vi "CODCr质控流程 (子VI).vi"(9 "CODCr量程切换":enum32{"H", "L", "AUTO"}(ring)=enum."AUTO", 10 "CODCr":bool) -> (3 "布尔":bool)   [LabVIEW 2016, in "质控单元.lvlib"]
panel:
  out "CODCr中断报警":bool
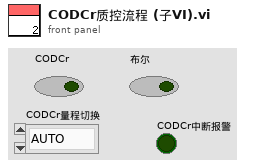
[diagram p1: front panel]
types:
  T1 = enum16{"待机", "启动水样测量", "水样测量中", "启动加标", "启动加标回收", "加标回收测量中", "结束"}
  T2 = cluster{"测量模式":enum16{"水样测量", "标样核查", "零点核查", "跨度核查", "空白测试", "加标回收", "平行样", "校零", "校标"}}
  T3 = enum16{"空闲", "水样测试", "标样核查", "零点核查", "跨度核查", "空白测试", "平行样测试", "加标回收", "空白校准", "标样校准", "初始化（清洗）"}
  T4 = cluster{"系统时间":timestamp, "工作状态":enum16{"空闲", "水样测试", "标样核查", "零点核查", "跨度核查", "空白测试", "平行样测试", "加标回收", "空白校准", "标样校准", "初始化（清洗）"}, "测量模式":enum16{"待机", "连续模式", "周期模式", "定点模式", "受控模式", "手动模式"}, "告警代码":enum16{"无告警", "缺试剂告警", "缺水样告警", "缺蒸馏水告警", "缺标液告警", "仪表漏液告警", "标定异常告警", "超量程告警", "加热异常", "低试剂预警", "超上限告警", "超下限告警", "仪表内部其他异常", "滴定异常告警", "电极异常告警", "量程切换告警", "参数设置告警", "PH电极电位异常", "电导率电极异常", "浊度光度异常", "溶解氧电极异常", "溶解氧光强异常", "温度异常告警", "PH异常告警", "溶解氧异常告警", "电导率异常告警", "浊度异常告警", "叶绿素异常告警", "藻密度异常告警", "蓝绿藻异常告警", "ORP异常告警", "氨氮异常告警", "清洁刷异常告警", "SD卡异常告警", "蓝牙异常告警", "Wifi异常告警", "流程异常告警"}, "故障代码":enum16{"无故障", "电机故障", "温度故障", "通讯故障", "滴定故障"}, "日志代码":u16, "软件版本":u16, "F0":sgl, "F1":sgl, "F2":sgl, "F3":sgl, "T":sgl, "H":sgl, "id":u16, "flowid":u16, "量程":u16, "总磷控温温度1":sgl, "营养盐控温温度2":sgl, "ADC":sgl}
  T5 = cluster{"因子编码":u32, "单位":u16, "标样参考值":sgl, "水样数据时间":timestamp, "水样实测值":sgl, "水样数据标识":string, "标样数据时间":timestamp, "标样实测值":sgl, "标样数据标识":string, "空白数据时间":timestamp, "空白实测值":sgl, "空白数据标识":string, "零点核查数据时间":timestamp, "零点核查实测值":sgl, "零点核查数据标识":string, "跨度核查数据时间":timestamp, "跨度核查实测值":sgl, "跨度核查数据标识":string, "加标回收数据时间":timestamp, "加标回收实测值":sgl, "加标回收数据标识":string, "平行样数据时间":timestamp, "平行样实测值":sgl, "平行样数据标识":string}
  T6 = cluster{"量程":dbl, "检出限":dbl, "加标前水样浓度":dbl, "加标后水样浓度":dbl, "加标水杯定容体积":dbl, "加标母液浓度":dbl, "加标体积":dbl, "加标回收率":dbl}
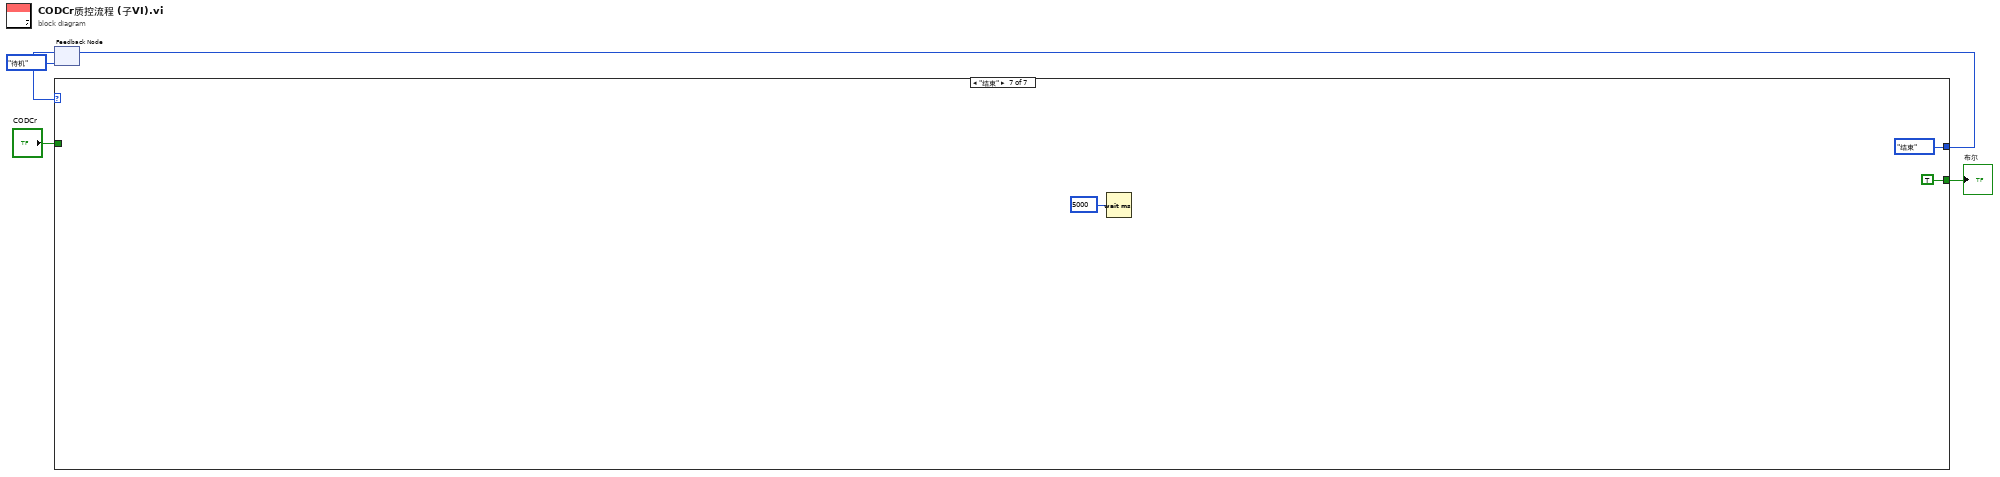
[diagram p0: block diagram]
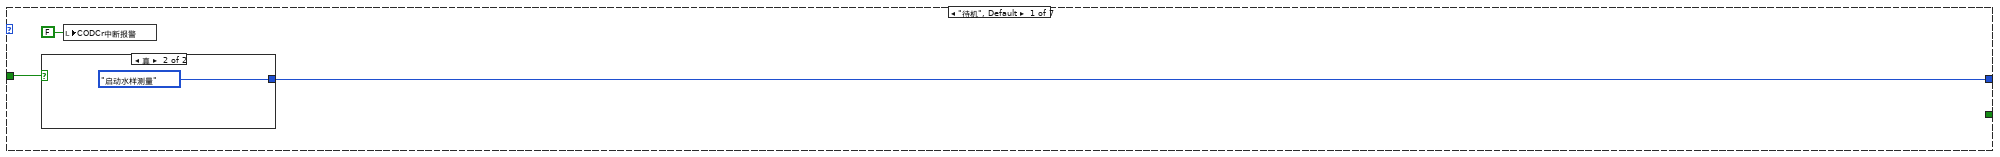
[diagram p2: hidden frame]
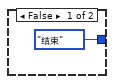
[diagram p3: hidden frame]
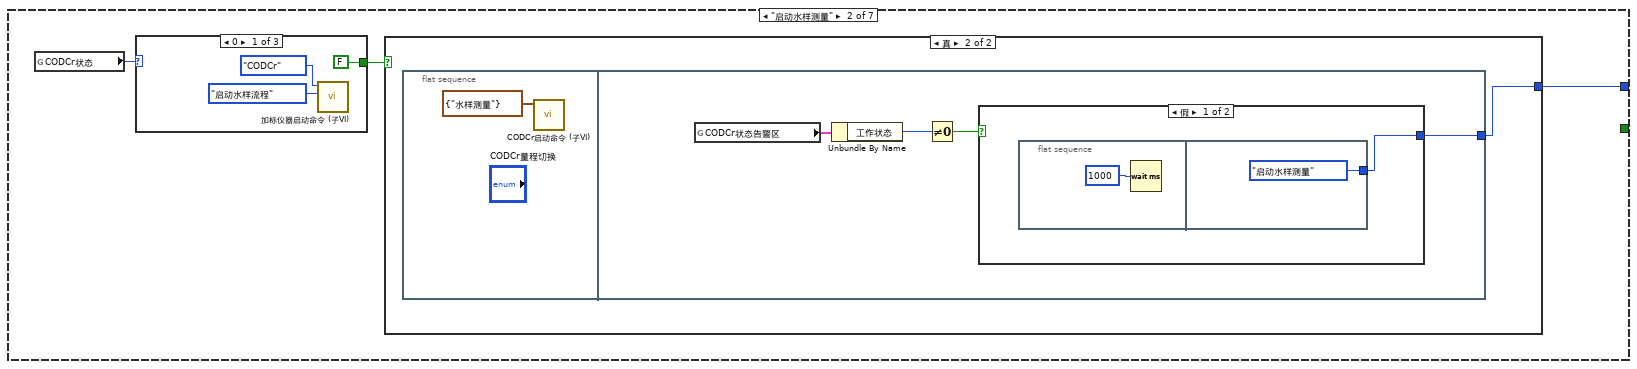
[diagram p4: hidden frame]
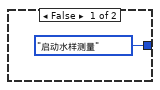
[diagram p5: hidden frame]
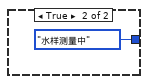
[diagram p6: hidden frame]
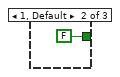
[diagram p7: hidden frame]
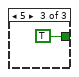
[diagram p8: hidden frame]
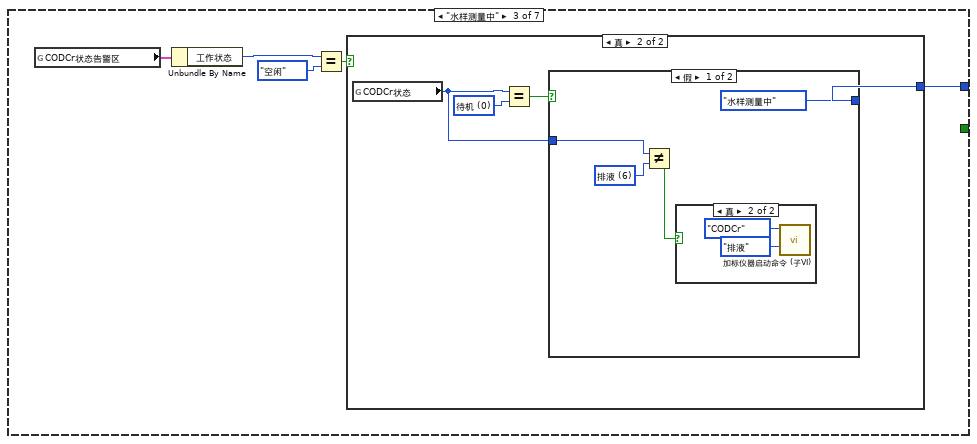
[diagram p9: hidden frame]
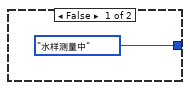
[diagram p10: hidden frame]
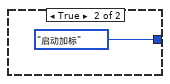
[diagram p12: hidden frame]
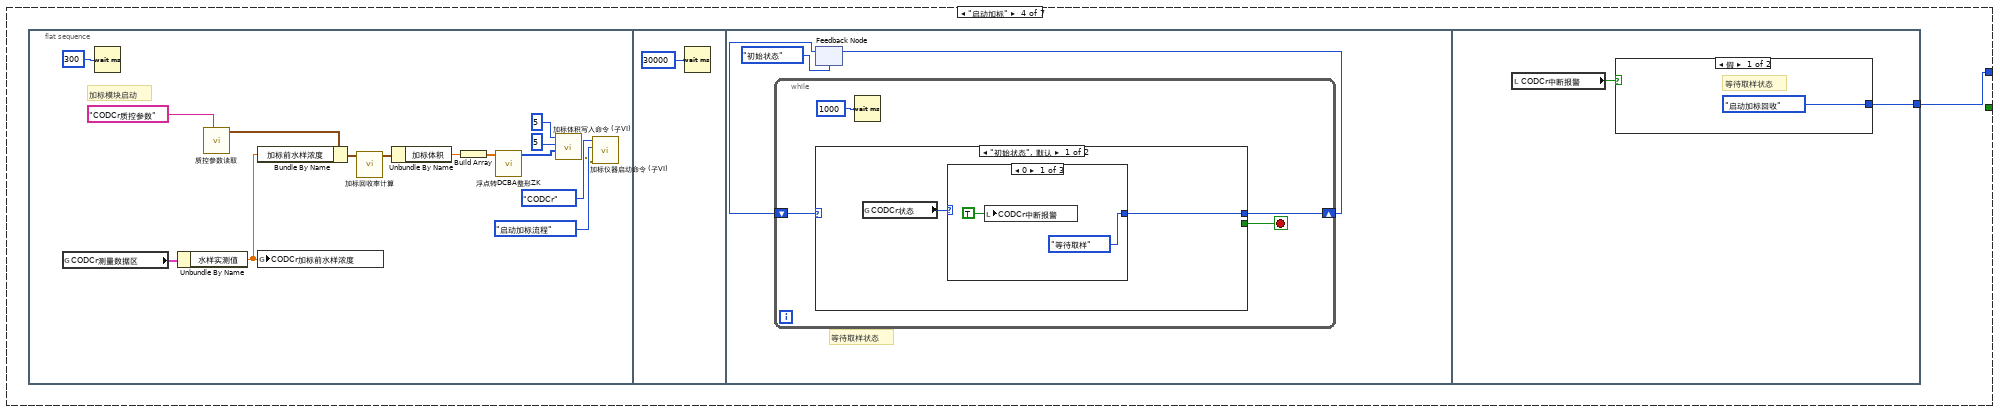
[diagram p13: hidden frame]
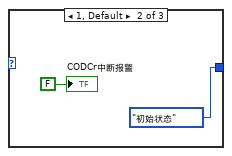
[diagram p14: hidden frame]
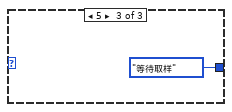
[diagram p15: hidden frame]
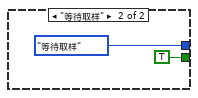
[diagram p16: hidden frame]
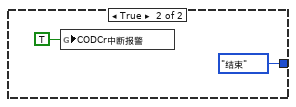
[diagram p17: hidden frame]
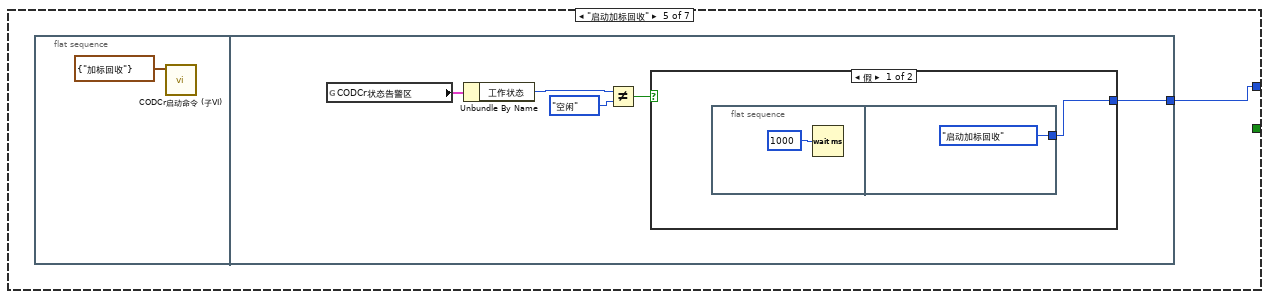
[diagram p18: hidden frame]
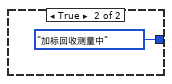
[diagram p19: hidden frame]
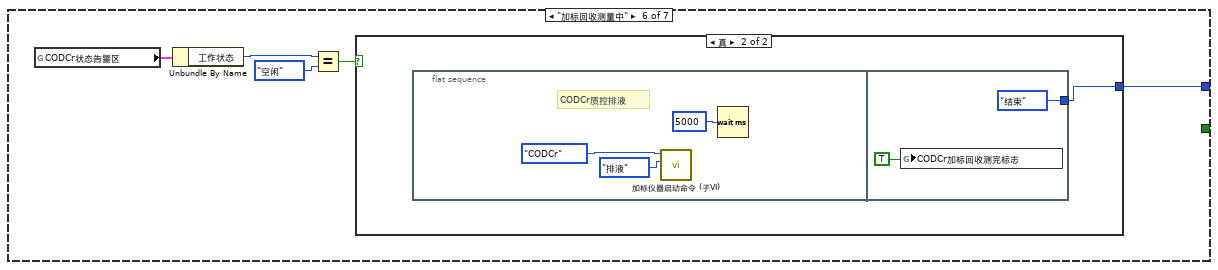
[diagram p20: hidden frame]
diagram:
  n1 = feedback #1(T1."待机") -> (w3:T1)
  n2 = case shown="\"结束\"" w3 {
    tunnel: [w8 w13 w34 w47 w85 w100 T1."结束"] -> w4
    tunnel: [_ _ _ _ _ _ TRUE] -> w2
    tunnel: "CODCr" -> [w7 _ _ _ _ _ _]
    frame "待机", Default {
      n3 = case shown="真" w7 {
        tunnel: [T1."结束" T1."启动水样测量"] -> w8
        frame False {
        }
        frame True {
        }
      }
      n4 = local write "CODCr中断报警"(FALSE ("CODMn中断报警")) -> ()
    }
    frame "启动水样测量" {
      n5 = global read "加标回收状态全局变量.vi" "CODCr状态"() -> (w12:u16)
      n6 = case shown="0" w12 {
        tunnel: [FALSE ("s") FALSE ("s") TRUE ("s")] -> w11
        frame 0 {
          n7 = call "加标仪器启动命令 (子VI).vi"("启动命令"=enum16{"启动水样流程", "启动加标流程", "排液", "停止"}."启动水样流程", "仪器"=enum16{"", "氨氮", "总磷", "总氮", "CODMn", "CODCr"}."CODCr") -> ()  [unwired: 9 in, 1 out]
        }
        frame 1, Default {
        }
        frame 5 {
        }
      }
      n8 = case shown="真" w11 {
        tunnel: [T1."启动水样测量" w15] -> w13
        frame False {
        }
        frame True {
          n9 = flat-sequence {
            tunnel: [w20] -> w15
            frame #0 {
              n10 = call "CODCr启动命令 (子VI).vi"("启动测量模式"=T2 {"测量模式"=enum."水样测量"}) -> ()  [unwired: 10 in, 1 out]
            }
            frame #1 {
              n11 = global read "与CODCr交互全局.vi" "CODCr状态告警区"() -> (w18:T4)
              n12 = Unbundle By Name(w18) -> ("工作状态"=w19:T3)
              n13 = Not Equal To 0?(x=w19) -> (x != 0?=w17:bool)
              n14 = case shown="假" w17 {
                tunnel: [w21 T1."水样测量中"] -> w20
                frame False {
                  n15 = flat-sequence {
                    tunnel: [T1."启动水样测量"] -> w21
                    frame #0 {
                      n16 = Wait (ms)(milliseconds to wait=u32 1000 ("等待时间（毫秒）")) -> ()  [unwired: 1 out]
                    }
                    frame #1 {
                    }
                  }
                }
                frame True {
                }
              }
            }
          }
        }
      }
    }
    frame "水样测量中" {
      n17 = global read "与CODCr交互全局.vi" "CODCr状态告警区"() -> (w31:T4)
      n18 = Unbundle By Name(w31) -> ("工作状态"=w30:T3)
      n19 = Equal?(x=w30, y=T3."空闲") -> (x = y?=w32:bool)
      n20 = case shown="真" w32 {
        tunnel: [T1."水样测量中" w39] -> w34
        frame False {
        }
        frame True {
          w38 = u16 0 items=["待机", "润洗", "进样", "进样完成", "柱塞泵加标", "等待取液", "排液"] ("CODCr状态")
          n21 = global read "加标回收状态全局变量.vi" "CODCr状态"() -> (w36:u16)
          n22 = Equal?(x=w36, y=w38) -> (x = y?=w37:bool)
          n23 = case shown="假" w37 {
            tunnel: [T1."水样测量中" T1."启动加标"] -> w39
            tunnel: w36 -> [w40 _]
            frame False {
              w42 = u16 6 items=["待机", "润洗", "进样", "进样完成", "柱塞泵加标", "等待取液", "排液"] ("氨氮状态")
              n24 = Not Equal?(x=w40, y=w42) -> (x != y?=w41:bool)
              n25 = case shown="真" w41 {
                frame False {
                }
                frame True {
                  n26 = call "加标仪器启动命令 (子VI).vi"("启动命令"=enum16{"启动水样流程", "启动加标流程", "排液", "停止"}."排液", "仪器"=enum16{"", "氨氮", "总磷", "总氮", "CODMn", "CODCr"}."CODCr") -> ()  [unwired: 9 in, 1 out]
                }
              }
            }
            frame True {
            }
          }
        }
      }
    }
    frame "启动加标" {
      n27 = flat-sequence {
        tunnel: [w81] -> w47
        frame #0 {
          # "加标模块启动"
          n28 = global read "与CODCr交互全局.vi" "CODCr测量数据区"() -> (w55:T5)
          n29 = Wait (ms)(milliseconds to wait=u32 300 ("等待时间（毫秒）")) -> ()  [unwired: 1 out]
          n30 = Unbundle By Name(w55) -> ("水样实测值"=w56:sgl)
          n31 = call "质控参数读取.vi"("section"="CODCr质控参数") -> ("参数"=w60:T6)  [unwired: 9 in, 1 out]
          n32 = Bundle By Name(cluster=w60, "加标前水样浓度"=w56) -> (w61:T6)
          n33 = global write "水样浓度全局.vi" "CODCr加标前水样浓度"(w56) -> ()
          n34 = call "加标回收率计算.vi"("参数"=w61) -> ("参数 out"=w59:T6)  [unwired: 9 in, 1 out]
          n35 = Unbundle By Name(w59) -> ("加标体积"=w58:dbl)
          n36 = Build Array(w58) -> (w54:dbl[])
          n37 = call "浮点转DCBA整形ZK.vi"("浮点数"=w54) -> ("DCBA整形输出"=w49:u16[])  [unwired: 10 in]
          n38 = call "加标体积写入命令 (子VI).vi"("values"=w49, "starting address"=u16 5, "Slave ID"=u16 5 ("value")) -> ("错误输出"=w48:errorcluster)  [unwired: 8 in]
          n39 = call "加标仪器启动命令 (子VI).vi"("错误输入（无错误）"=w48, "启动命令"=enum16{"启动水样流程", "启动加标流程", "排液", "停止"}."启动加标流程", "仪器"=enum16{"", "氨氮", "总磷", "总氮", "CODMn", "CODCr"}."CODCr") -> ()  [unwired: 8 in, 1 out]
        }
        frame #1 {
          n40 = Wait (ms)(milliseconds to wait=u32 30000 ("等待时间（毫秒）")) -> ()  [unwired: 1 out]
        }
        frame #2 {
          # "等待取样状态"
          n41 = feedback #2(enum16{"初始状态", "等待取样"}."初始状态") -> (w65:enum16{"初始状态", "等待取样"})
          n42 = while {
            shift-right: [w69] -> w66
            shift-left: w65 -> [w70]
            stop <- w68 stop-if-true
            n43 = case shown="\"初始状态\", 默认" w70 {
              tunnel: [w72 enum16{"初始状态", "等待取样"}."等待取样"] -> w69
              tunnel: [_ TRUE] -> w68
              frame "初始状态", Default {
                n44 = global read "加标回收状态全局变量.vi" "CODCr状态"() -> (w71:u16)
                n45 = case shown="0" w71 {
                  tunnel: [enum16{"初始状态", "等待取样"}."等待取样" enum16{"初始状态", "等待取样"}."初始状态" enum16{"初始状态", "等待取样"}."等待取样"] -> w72
                  frame 0 {
                    n46 = local write "CODCr中断报警"(TRUE ("氨氮中断报警")) -> ()
                  }
                  frame 1, Default {
                    "CODCr中断报警" <- FALSE ("总氮中断报警")
                  }
                  frame 5 {
                  }
                }
              }
              frame "等待取样" {
              }
            }
            n47 = Wait (ms)(milliseconds to wait=u32 1000 ("等待时间（毫秒）")) -> ()  [unwired: 1 out]
          }
          n48 = feedback-in #2(w66) -> ()
        }
        frame #3 {
          n49 = local read "CODCr中断报警"() -> (w80:bool)
          n50 = case shown="假" w80 {
            tunnel: [T1."启动加标回收" T1."结束"] -> w81
            frame False {
              # "等待取样状态"
            }
            frame True {
              n51 = global write "质控中断报警全局.vi" "CODCr中断报警"(TRUE ("CODCr中断报警")) -> ()
            }
          }
        }
      }
    }
    frame "启动加标回收" {
      n52 = flat-sequence {
        tunnel: [w91] -> w85
        frame #0 {
          n53 = call "CODCr启动命令 (子VI).vi"("启动测量模式"=T2 {"测量模式"=enum."加标回收"}) -> ()  [unwired: 10 in, 1 out]
        }
        frame #1 {
          n54 = global read "与CODCr交互全局.vi" "CODCr状态告警区"() -> (w90:T4)
          n55 = Unbundle By Name(w90) -> ("工作状态"=w89:T3)
          n56 = Not Equal?(x=w89, y=T3."空闲") -> (x != y?=w87:bool)
          n57 = case shown="假" w87 {
            tunnel: [w92 T1."加标回收测量中"] -> w91
            frame False {
              n58 = flat-sequence {
                tunnel: [T1."启动加标回收"] -> w92
                frame #0 {
                  n59 = Wait (ms)(milliseconds to wait=u32 1000 ("等待时间（毫秒）")) -> ()  [unwired: 1 out]
                }
                frame #1 {
                }
              }
            }
            frame True {
            }
          }
        }
      }
    }
    frame "加标回收测量中" {
      n60 = global read "与CODCr交互全局.vi" "CODCr状态告警区"() -> (w97:T4)
      n61 = Unbundle By Name(w97) -> ("工作状态"=w96:T3)
      n62 = Equal?(x=w96, y=T3."空闲") -> (x = y?=w98:bool)
      n63 = case shown="真" w98 {
        tunnel: [T1."加标回收测量中" w102] -> w100
        frame False {
        }
        frame True {
          n64 = flat-sequence {
            tunnel: [T1."结束"] -> w102
            frame #0 {
              # "CODCr质控排液"
              n65 = call "加标仪器启动命令 (子VI).vi"("启动命令"=enum16{"启动水样流程", "启动加标流程", "排液", "停止"}."排液", "仪器"=enum16{"", "氨氮", "总磷", "总氮", "CODMn", "CODCr"}."CODCr") -> ()  [unwired: 9 in, 1 out]
              n66 = Wait (ms)(milliseconds to wait=u32 5000 ("等待时间（毫秒）")) -> ()  [unwired: 1 out]
            }
            frame #1 {
              n67 = global write "质控测完标志全局 1.vi" "CODCr加标回收测完标志"(TRUE ("COD加标回收测完标志")) -> ()
            }
          }
        }
      }
    }
    frame "结束" {
      n68 = Wait (ms)(milliseconds to wait=u32 5000 ("等待时间（毫秒）")) -> ()  [unwired: 1 out]
    }
  }
  "布尔" <- w2
  n69 = feedback-in #1(w4) -> ()
